vi "Advanced_PID_Example.vi"() -> ()   [LabVIEW 2019]
uses:
  <vilib>/Rock Robotics/WPI/ThirdParty/JAS_Junk/TrajLib/Trajectory_Library.lvlib
  <vilib>/Rock Robotics/WPI/ThirdParty/JAS_Junk/TrajLib/LinearFilter_MovingAvg_Execute.vi
  <vilib>/Rock Robotics/WPI/ThirdParty/JAS_Junk/TrajLib/TypeDef/PID_CONTROLLER.ctl
  <vilib>/Rock Robotics/WPI/ThirdParty/JAS_Junk/TrajLib/TypeDef/PID_ADV_TUNING.ctl
panel:
  in  "Desired Speed":dbl(slide)=-0.22222222222222499 scale=-50.0..50.0 scale format="%#.1f"
  in  "Tab Control":T1(tab)
  in  "Enable Noise":bool=TRUE
  in  "Auto / Manual":bool=TRUE
  out "Dash Speed Demand":dbl format="%10.2f"
  out "Dash Speed Target":dbl format="%10.2f"
  out "DashRightMotorOutput":dbl format="%11.3f"
  out "DashRight Wheel Speed":dbl(knob)=-2.895988890827539e-05 scale=-60.0..60.0
  out "Right Wheel ErrorFilt":dbl format="%11.3f"
  out "Right Wheel SpeedFilt":dbl format="%10.2f"
  out "DashLeft Wheel Speed":dbl(knob)=-2.895988890827539e-05 scale=-60.0..60.0
  out "Left Wheel ErrorFilt":dbl format="%11.3f"
  out "DashLeftMotorOutput":dbl format="%11.3f"
  out "Left Wheel Speed Filt":dbl format="%10.2f"
  out "Duration":dbl format="%11.3f"
  out "Late":dbl format="%11.3f"
  out "Auto":bool
  out "SP, PV, CO Left":T2(graph)
  out "SP, PV, CO Right":T2(graph)
  in  "Right Adv PID Tuning":T3={"Kf"=0.02, "Kp"=0.2, "Ki"=0.35, "Kd"=0.004, "MaximumIntegral"=9.9e+30, "MinimumIntegral"=-9.9e+30, "Filter Derivative"=TRUE, "IntegralZone"=8.0}
  in  "SetPoint Change Rate":dbl=80.0 min=1.0 max=9000.0 format="%14.4f"
  in  "Right PID Error Tolerance":T4={"PositionTolerance"=0.001, "VelocityTolerance"=9.9e+30}
  in  "Right Adv PID Limits":T5={"MaxInput"=50.0, "MinInput"=-50.0, "Continuous"=FALSE, "MaxOutput"=1.0, "MinOutput"=-1.0}
  in  "Left Adv PID Limits":T5={"MaxInput"=50.0, "MinInput"=-50.0, "Continuous"=FALSE, "MaxOutput"=1.0, "MinOutput"=-1.0}
  in  "Left PID Error Tolerance":T4={"PositionTolerance"=0.001, "VelocityTolerance"=9.9e+30}
  in  "Left Adv PID Tuning":T3={"Kf"=0.02, "Kp"=0.2, "Ki"=0.35, "Kd"=0.004, "MaximumIntegral"=9.9e+30, "MinimumIntegral"=-9.9e+30, "Filter Derivative"=TRUE, "IntegralZone"=8.0}
  out "Left PID Data":T6={"Kp"=0.0, "Ki"=0.0, "Kd"=0.0, "Period"=0.0, "Max_Integral"=0.0, "Min_Integral"=0.0, "Max_Input"=0.0, "Min_Input"=0.0, "Continuous"=FALSE, "PositionError"=0.0, "VelocityError"=0.0, "PrevError"=0.0, "Total_Integral"=0.0, "PositionTolerance"=0.0, "VelocityTolerance"=0.0, "SetPoint"=0.0, "Kf"=0.0, "Prev_Deriv"=0.0, "Prev_Deriv 2"=0.0, "DerivativeFilter"=FALSE, "Min_Output"=-9.99e+35, "Max_Output"=9.9e+35, "Prev_F_P"=0.0, "Prev_F_P_2"=0.0, "AntiWindupActive"=FALSE, "Measurement"=0.0, "IntegralZone"=9.9e+30} {"IntegralZone" format="%16_6e"; "Measurement" format="%16_6e"; "Prev_F_P_2" format="%16_6e"; "Prev_F_P" format="%16_6e"; "Max_Output" format="%16_6e"; "Min_Output" format="%16_6e"; "Prev_Deriv 2" format="%16_6e"; "Prev_Deriv" format="%16_6e"; "Kf" format="%16_6e"; "SetPoint" format="%16_6e"; "VelocityTolerance" format="%16_6e"; "PositionTolerance" format="%16_6e"; "Total_Integral" format="%16_6e"; "PrevError" format="%16_6e"; "VelocityError" format="%16_6e"; "PositionError" format="%16_6e"; "Min_Input" format="%16_6e"; "Max_Input" format="%16_6e"; "Min_Integral" format="%16_6e"; "Max_Integral" format="%16_6e"; "Period" format="%16_6e"; "Kd" format="%16_6e"; "Ki" format="%16_6e"; "Kp" format="%16_6e"}
  out "Right PID Data":T6={"Kp"=0.0, "Ki"=0.0, "Kd"=0.0, "Period"=0.0, "Max_Integral"=0.0, "Min_Integral"=0.0, "Max_Input"=0.0, "Min_Input"=0.0, "Continuous"=FALSE, "PositionError"=0.0, "VelocityError"=0.0, "PrevError"=0.0, "Total_Integral"=0.0, "PositionTolerance"=0.0, "VelocityTolerance"=0.0, "SetPoint"=0.0, "Kf"=0.0, "Prev_Deriv"=0.0, "Prev_Deriv 2"=0.0, "DerivativeFilter"=FALSE, "Min_Output"=-9.99e+35, "Max_Output"=9.9e+35, "Prev_F_P"=0.0, "Prev_F_P_2"=0.0, "AntiWindupActive"=FALSE, "Measurement"=0.0, "IntegralZone"=9.9e+30} {"IntegralZone" format="%16_6e"; "Measurement" format="%16_6e"; "Prev_F_P_2" format="%16_6e"; "Prev_F_P" format="%16_6e"; "Max_Output" format="%16_6e"; "Min_Output" format="%16_6e"; "Prev_Deriv 2" format="%16_6e"; "Prev_Deriv" format="%16_6e"; "Kf" format="%16_6e"; "SetPoint" format="%16_6e"; "VelocityTolerance" format="%16_6e"; "PositionTolerance" format="%16_6e"; "Total_Integral" format="%16_6e"; "PrevError" format="%16_6e"; "VelocityError" format="%16_6e"; "PositionError" format="%16_6e"; "Min_Input" format="%16_6e"; "Max_Input" format="%16_6e"; "Min_Integral" format="%16_6e"; "Max_Integral" format="%16_6e"; "Period" format="%16_6e"; "Kd" format="%16_6e"; "Ki" format="%16_6e"; "Kp" format="%16_6e"}
  out "RightWheelSpeed":dbl
  out "LeftWheelSpeed":dbl
  out "RightMotorOutput":dbl
  out "LeftMotorOutput":dbl
  out "SpeedSetpoint":dbl
  out "LibUsage_Kinematics":i32 format="%20.0f"
  out "LibUsage_TrapezoidProfile":i32 format="%20.0f"
  out "LibUsage_LinearFIlter":i32 format="%20.0f"
  out "LibUsage_Odometry":i32 format="%20.0f"
  out "LibUsage_PIDController":i32 format="%20.0f"
  out "LibUsage_ProfiledPID":i32 format="%20.0f"
  # "Enter a desired speed and then press the Set Speed Target \nbutton.  This simulates the joystick input."
  # "Advanced PID Example - Simple Simulated Drive"
  # "FT/SEC"
  # "This value shows the current speed of each wheel.  This is measured by an encoder.  The encoder measures\n speed by counting pulses of the wheel turning and dividing by the time interval.  Total distance change\nis also a result.  This value is called the \"Process Variable\"."
  # "FT/SEC"
  # "FT/SEC"
  # "FT/SEC"
  # "The Speed Target is rate limited so not to make\nto drastic a change in the desired speed.  (This is\nwhat happens mechanically when pushing the gas\npedal of a real car.)"
  # "This error value shows the error between the current speed\nand the speed demand."
  # "FT/SEC"
  # "This example adds a \"Manual\" mode so that the still operates\nif the encoder fails."
  # "FT/SEC"
  # "FT/SEC"
  # "This value shows the current motor output demand.  This could also be a motor speed demand and \nanother closed loop controller would control the motor speed.  In this simple example this value is \nused to drive the simulated motor directly.  This motor demand is called the \"Control Output\"."
  # "Enables some simulated process noise"
  # "FT/SEC/SEC"
  # "These are the tuning parameters for the PID VI"
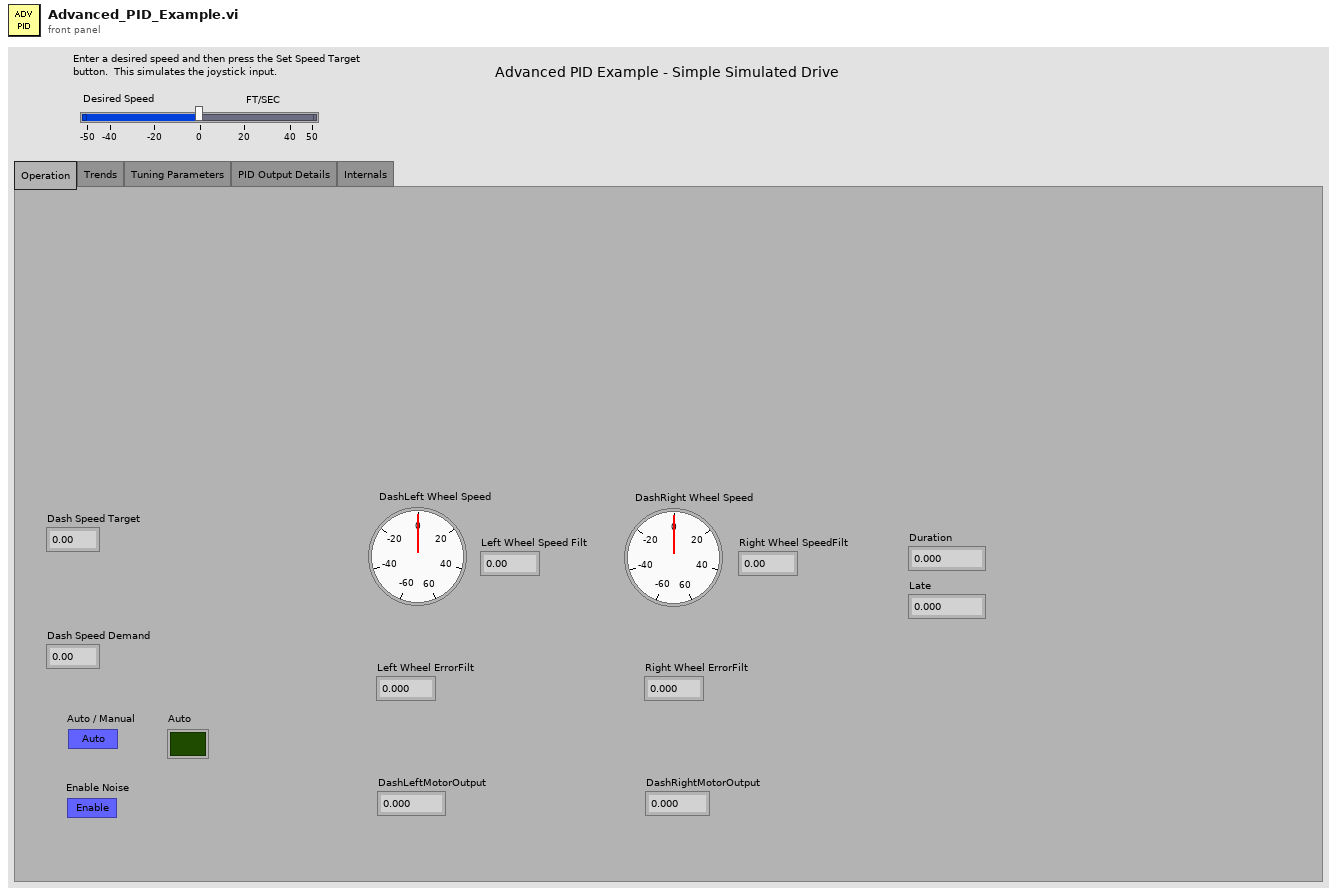
[diagram p1: front panel]
types:
  T1 = enum32{"Operation", "Trends", "Tuning Parameters", "PID Output Details", "Internals"}
  T2 = cluster{"MotorDemand":dbl, "CurrentSetpoint":dbl, "CurrentPosition":dbl}
  T3 = typedef "Trajectory_Library.lvlib/PID_ADV_TUNING.ctl" = cluster{"Kf":dbl, "Kp":dbl, "Ki":dbl, "Kd":dbl, "MaximumIntegral":dbl, "MinimumIntegral":dbl, "Filter Derivative":bool, "IntegralZone":dbl}
  T4 = cluster{"PositionTolerance":dbl, "VelocityTolerance":dbl}
  T5 = cluster{"MaxInput":dbl, "MinInput":dbl, "Continuous":bool, "MaxOutput":dbl, "MinOutput":dbl}
  T6 = typedef "Trajectory_Library.lvlib/PID_CONTROLLER.ctl" = cluster{"Kp":dbl, "Ki":dbl, "Kd":dbl, "Period":dbl, "Max_Integral":dbl, "Min_Integral":dbl, "Max_Input":dbl, "Min_Input":dbl, "Continuous":bool, "PositionError":dbl, "VelocityError":dbl, "PrevError":dbl, "Total_Integral":dbl, "PositionTolerance":dbl, "VelocityTolerance":dbl, "SetPoint":dbl, "Kf":dbl, "Prev_Deriv":dbl, "Prev_Deriv 2":dbl, "DerivativeFilter":bool, "Min_Output":dbl, "Max_Output":dbl, "Prev_F_P":dbl, "Prev_F_P_2":dbl, "AntiWindupActive":bool, "Measurement":dbl, "IntegralZone":dbl}
  T7 = cluster{"LeftMotorOutput":dbl, "SpeedSetpoint":dbl, "LeftWheelSpeed":dbl}
  T8 = cluster{"RightMotorOutput":dbl, "SpeedSetpoint":dbl, "RightWheelSpeed":dbl}
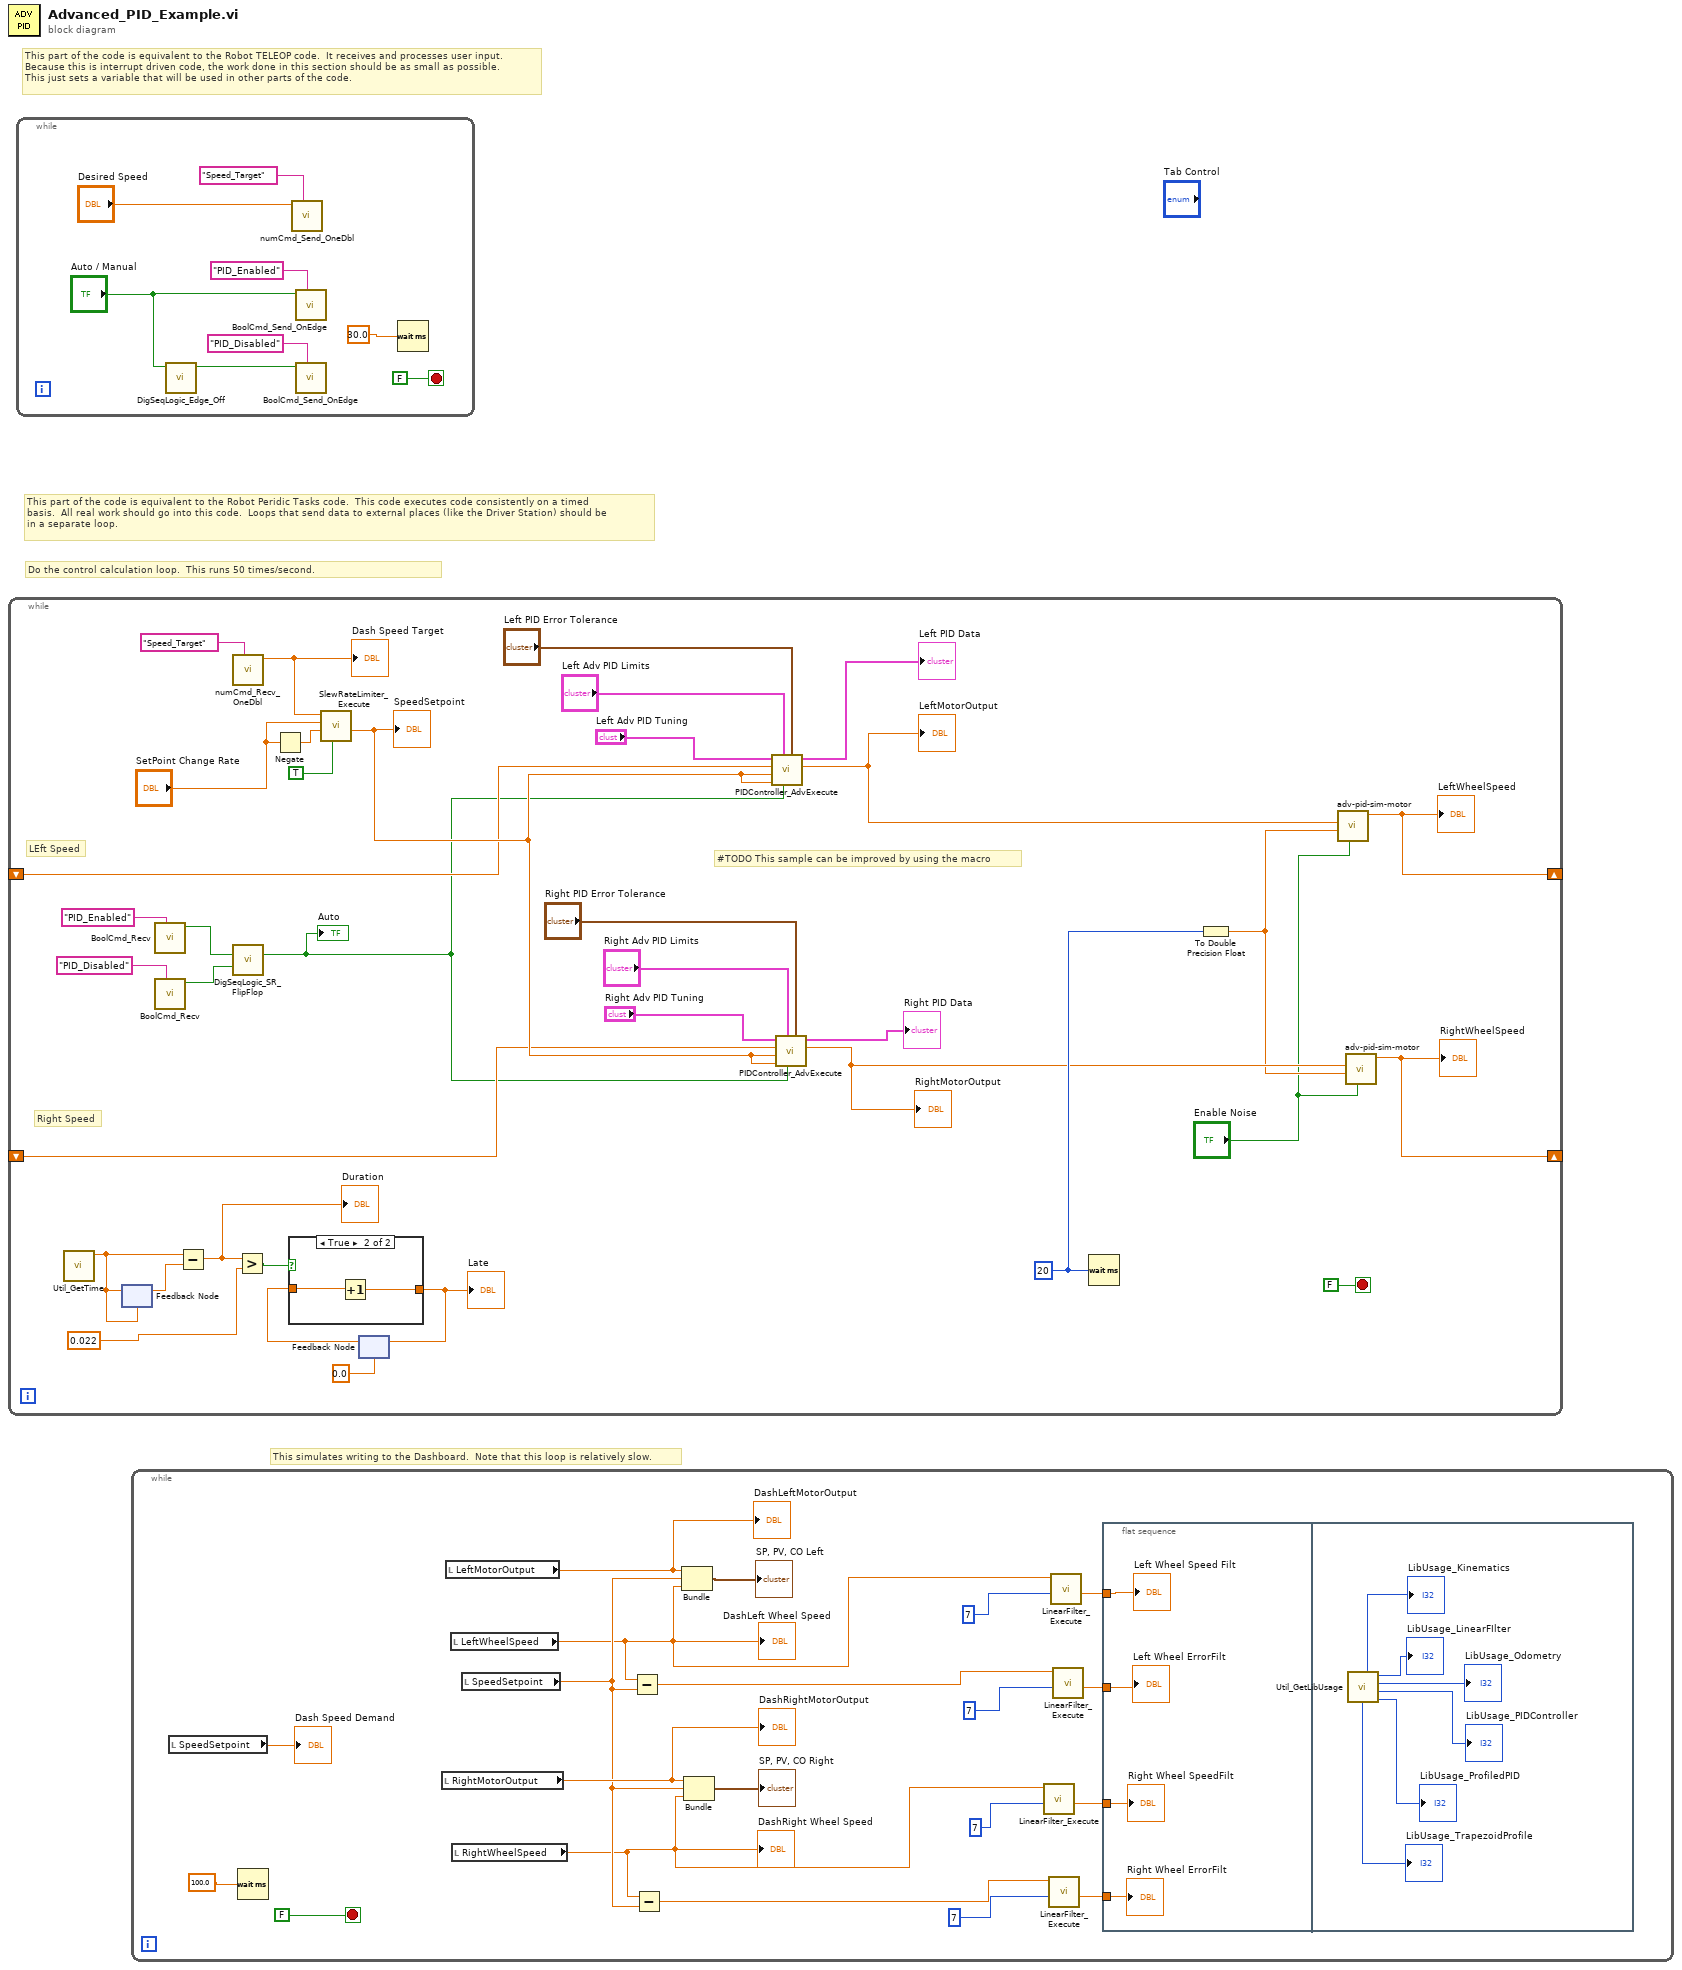
[diagram p0: block diagram]
diagram:
  # "This simulates writing to the Dashboard.  Note that this loop is relatively slow."
  # "Do the control calculation loop.  This runs 50 times/second."
  # "This part of the code is equivalent to the Robot Peridic Tasks code.  This code executes code consistently on a timed\nbasis.  All real work should go into this code.  Loops that send data to external places (like the Driver Station) should be \nin a separate loop."
  # "This part of the code is equivalent to the Robot TELEOP code.  It receives and processes user input.\nBecause this is interrupt driven code, the work done in this section should be as small as possible.\nThis just sets a variable that will be used in other parts of the code."
  n1 = while {
    shift-right: [w14] -> _
    shift-left: _ -> [w12]
    shift-right: [w13] -> _
    shift-left: _ -> [w11]
    stop <- FALSE stop-if-true
    w26 = u32 20 ("milliseconds to wait")
    # "#TODO This sample can be improved by using the macro"
    # "Right Speed"
    # "LEft Speed"
    n2 = call <vilib>:"Util_GetTime.vi"() -> ("FPGA_Time_Seconds"=w32:dbl)  [unwired: 9 in, 2 out]
    n3 = feedback #1(w32) -> (w31:dbl)
    n4 = feedback-in #1(w32) -> ()
    n5 = call <vilib>:"BoolCmd_Recv.vi"("Command Name"="PID_Enabled") -> ("New Request"=w9:bool)  [unwired: 9 in, 1 out]
    n6 = call <vilib>:"BoolCmd_Recv.vi"("Command Name"="PID_Disabled") -> ("New Request"=w8:bool)  [unwired: 9 in, 1 out]
    n7 = Subtract(x=w32, y=w31) -> (x-y=w29:dbl)
    "Duration" <- w29
    n8 = call <vilib>:"numCmd_Recv_OneDbl.vi"("Command Name"="Speed_Target") -> ("Value"=w3:dbl)  [unwired: 8 in, 2 out]
    "Dash Speed Target" <- w3
    n9 = call <vilib>:"DigSeqLogic_SR_FlipFlop.vi"("Set"=w9, "Reset"=w8) -> ("Output"=w5:bool)  [unwired: 12 in, 1 out]
    "Auto" <- w5
    n10 = Greater?(x=w29, y=0.022) -> (0:w30:bool)
    n11 = Negate(x="SetPoint Change Rate") -> (-x=w17:dbl)
    n12 = call <vilib>:"SlewRateLimiter_Execute.vi"("Enable"=TRUE, "NegativeRate"=w17, "PositiveRate"="SetPoint Change Rate", "Input"=w3) -> ("Output"=w23:dbl)  [unwired: 6 in, 1 out]
    "SpeedSetpoint" <- w23
    n13 = feedback #2(0.0) -> (w33:dbl)
    n14 = case shown="True" w30 {
      tunnel: [w38 w40] -> w34
      tunnel: w33 -> [w38 w39]
      frame False {
      }
      frame True {
        n15 = Increment(x=w39) -> (x+1=w40:dbl)
      }
    }
    "Late" <- w34
    n16 = feedback-in #2(w34) -> ()
    n17 = call <vilib>:"PIDController_AdvExecute.vi"("PID Error Tolerance"="Left PID Error Tolerance", "Auto"=w5, "Adv PID Limits"="Left Adv PID Limits", "FF-FeedForward"=w23, "SP-SetPoint"=w23, "PV-Measurement"=w12, "Adv PID Tuning"="Left Adv PID Tuning") -> ("CO-ControlOutput"=w20:dbl, "out PID_CONTROLLER"=→"Left PID Data":T6)  [unwired: 2 in, 1 out]
    "LeftMotorOutput" <- w20
    n18 = call <vilib>:"PIDController_AdvExecute.vi"("PID Error Tolerance"="Right PID Error Tolerance", "Auto"=w5, "Adv PID Limits"="Right Adv PID Limits", "FF-FeedForward"=w23, "SP-SetPoint"=w23, "PV-Measurement"=w11, "Adv PID Tuning"="Right Adv PID Tuning") -> ("CO-ControlOutput"=w16:dbl, "out PID_CONTROLLER"=→"Right PID Data":T6)  [unwired: 2 in, 1 out]
    "RightMotorOutput" <- w16
    n19 = Wait (ms)(milliseconds to wait=w26) -> ()  [unwired: 1 out]
    n20 = To Double Precision Float(number=w26) -> (double precision float=w15:dbl)
    n21 = call "adv-pid-sim-motor.vi"("Use Noise"="Enable Noise", "Cycle Time"=w15, "CO-ControlOutput"=w20) -> ("Motor Speed"=w14:dbl)  [unwired: 8 in]
    "LeftWheelSpeed" <- w14
    n22 = call "adv-pid-sim-motor.vi"("Use Noise"="Enable Noise", "Cycle Time"=w15, "CO-ControlOutput"=w16) -> ("Motor Speed"=w13:dbl)  [unwired: 8 in]
    "RightWheelSpeed" <- w13
  }
  n23 = while {
    stop <- FALSE stop-if-true
    n24 = call <vilib>:"DigSeqLogic_Edge_Off.vi"("Input"="Auto / Manual") -> ("Off Edge"=w44:bool)  [unwired: 10 in]
    n25 = call <vilib>:"numCmd_Send_OneDbl.vi"("Command Name"="Speed_Target", "Value"="Desired Speed") -> ()  [unwired: 9 in, 1 out]
    n26 = call <vilib>:"BoolCmd_Send_OnEdge.vi"("Command Name"="PID_Enabled", "Value"="Auto / Manual") -> ()  [unwired: 9 in, 1 out]
    n27 = call <vilib>:"BoolCmd_Send_OnEdge.vi"("Command Name"="PID_Disabled", "Value"=w44) -> ()  [unwired: 9 in, 1 out]
    n28 = Wait (ms)(milliseconds to wait=30.0) -> ()  [unwired: 1 out]
  }
  n29 = while {
    stop <- FALSE stop-if-true
    n30 = local read "SpeedSetpoint"() -> (→"Dash Speed Demand":dbl)
    n31 = Wait (ms)(milliseconds to wait=100.0) -> ()  [unwired: 1 out]
    n32 = local read "RightMotorOutput"() -> (w64:dbl)
    "DashRightMotorOutput" <- w64
    n33 = local read "LeftMotorOutput"() -> (w62:dbl)
    "DashLeftMotorOutput" <- w62
    n34 = local read "LeftWheelSpeed"() -> (w59:dbl)
    "DashLeft Wheel Speed" <- w59
    n35 = local read "RightWheelSpeed"() -> (w52:dbl)
    "DashRight Wheel Speed" <- w52
    n36 = local read "SpeedSetpoint"() -> (w61:dbl)
    n37 = Subtract(x=w59, y=w61) -> (x-y=w56:dbl)
    n38 = Subtract(x=w52, y=w61) -> (x-y=w50:dbl)
    n39 = Bundle("LeftMotorOutput"=w62, "SpeedSetpoint"=w61, "LeftWheelSpeed"=w59) -> (→"SP, PV, CO Left":T7)  [unwired: 1 in]
    n40 = Bundle("RightMotorOutput"=w64, "SpeedSetpoint"=w61, "RightWheelSpeed"=w52) -> (→"SP, PV, CO Right":T8)  [unwired: 1 in]
    n41 = call-poly <vilib>:"LinearFilter_Execute.vi"("Samples"=7, "Input"=w52) -> ("Output"=w53:dbl)  [unwired: 9 in]
    n42 = call-poly <vilib>:"LinearFilter_Execute.vi"("Samples"=7, "Input"=w50) -> ("Output"=w51:dbl)  [unwired: 9 in]
    n43 = call-poly <vilib>:"LinearFilter_Execute.vi"("Samples"=7, "Input"=w59) -> ("Output"=w58:dbl)  [unwired: 9 in]
    n44 = call-poly <vilib>:"LinearFilter_Execute.vi"("Samples"=7, "Input"=w56) -> ("Output"=w55:dbl)  [unwired: 9 in]
    n45 = flat-sequence {
      tunnel: w58 -> [w72]
      tunnel: w55 -> [w71]
      tunnel: w53 -> [w70]
      tunnel: w51 -> [w69]
      frame #0 {
        "Left Wheel ErrorFilt" <- w71
        "Right Wheel ErrorFilt" <- w69
        "Left Wheel Speed Filt" <- w72
        "Right Wheel SpeedFilt" <- w70
      }
      frame #1 {
        n46 = call <vilib>:"Util_GetLibUsage.vi"() -> ("LibUsage_ProfiledPID"=→"LibUsage_ProfiledPID":i32, "LibUsage_PIDController"=→"LibUsage_PIDController":i32, "LibUsage_Odometry"=→"LibUsage_Odometry":i32, "LibUsage_LinearFIlter"=→"LibUsage_LinearFIlter":i32, "LibUsage_TrapezoidProfile"=→"LibUsage_TrapezoidProfile":i32, "LibUsage_Kinematics"=→"LibUsage_Kinematics":i32)  [unwired: 6 in]
      }
    }
  }
